vi "Adc Conversion.vi"(8 "Error In":errorcluster, 10 "Numeric":dbl, 11 "Channel 2 In":refnum<class "Channel 2.lvclass">) -> (0 "Error Out":errorcluster, 2 "Channel Data":T1, 3 "Channel 2 Out":refnum<class "Channel 2.lvclass">)   [LabVIEW 2021, in "Channel 2.lvclass"]
doc: "This VI is an overriding method of channel 2 which performs the analog to digital conversion of channel 2 and stores it in U8 array."
uses:
  Channel 2.lvclass
  Controls/Channel Data.ctl
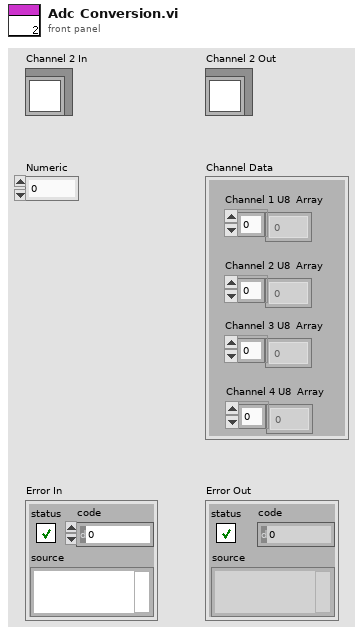
[diagram p1: front panel]
types:
  T1 = typedef "Channel Data.ctl" = cluster{"Channel 1 U8  Array":u8[], "Channel 2 U8  Array ":u8[], "Channel 3 U8  Array":u8[], "Channel 4 U8  Array":u8[]}
  T2 = typedef "ADC Type.ctl" = cluster{"Channels":string, "Range":dbl, "Resolution":dbl, "Sampling Rate":dbl}
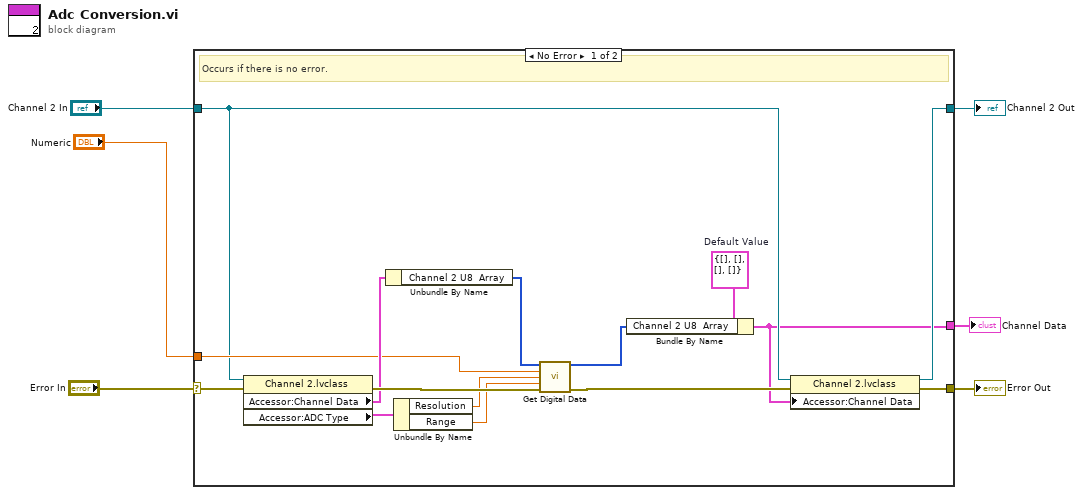
[diagram p0: block diagram]
diagram:
  n1 = case shown="No Error" "Error In" {
    selector: "Error In" -> [w21 w23]
    tunnel: [w12 w23] -> w5
    tunnel: [w10 w22] -> w3
    tunnel: "Channel 2 In" -> [w11 w22]
    tunnel: "Numeric" -> [w16 _]
    tunnel: [w7 _] -> w1
    frame No Error {
      w9 = T1 {"Channel 1 U8  Array"=[], "Channel 2 U8  Array "=[], "Channel 3 U8  Array"=[], "Channel 4 U8  Array"=[]}  # Default Value
      # "Occurs if there is no error."
      n2 = property class="Channel 2.lvclass"(reference=w11, error in=w21) -> (error out=w19:errorcluster, "Accessor:Channel Data"=w18:T1, "Accessor:ADC Type"=w15:T2)  [unwired: 1 out]
      n3 = Unbundle By Name(w18) -> ("Channel 2 U8  Array"=w17:u8[])
      n4 = Unbundle By Name(w15) -> ("Resolution"=w14:dbl, "Range"=w13:dbl)
      n5 = call "Get Digital Data.vi"("Input Array"=w17, "Analog Input"=w16, "Resolution"=w14, "Range"=w13, "Error In"=w19) -> ("Output Array"=w8:u8[], "Error Out"=w20:errorcluster)  [unwired: 9 in]
      n6 = Bundle By Name(cluster=w9, "Channel 2 U8  Array"=w8) -> (w7:T1)
      n7 = property class="Channel 2.lvclass"(reference=w11, error in=w20, "Accessor:Channel Data"=w7) -> (reference out=w10:refnum<class "Channel 2.lvclass">, error out=w12:errorcluster)
    }
    frame Error {
      # "Occurs if there is any error."
    }
  }
  "Error Out" <- w5
  "Channel 2 Out" <- w3
  "Channel Data" <- w1
